vi "Compare Configs.vi"(10 "Old Config":path, 11 "New Config":path) -> (3 "Time":dbl)   [LabVIEW 2015]
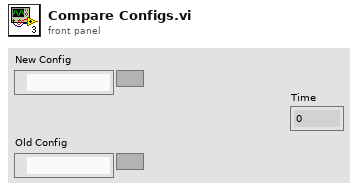
[diagram p1: front panel]
types:
  T1 = typedef "configuration.ctl" = cluster{"Primary Filter":string, "Secondary Filter":string, "Slit Mask":string, "Grating":string, "CS Target":dbl, "GS Target":dbl, "Coll Focus":i32, "Camera Focus":i32, "Name":string, "User":string, "Date":string, "Comment":string, "use Flexure Comp?":bool, "Select Mode:":u16}
  T2 = cluster{"Primary Filter":bool, "Secondary Filter":bool, "Slit Mask":bool, "Grating":bool, "CS Target":bool, "GS Target":bool, "Coll Focus":bool, "Camera Focus":bool, "Name":bool, "User":bool, "Date":bool, "Comment":bool, "use Flexure Comp?":bool, "Select Mode:":bool}
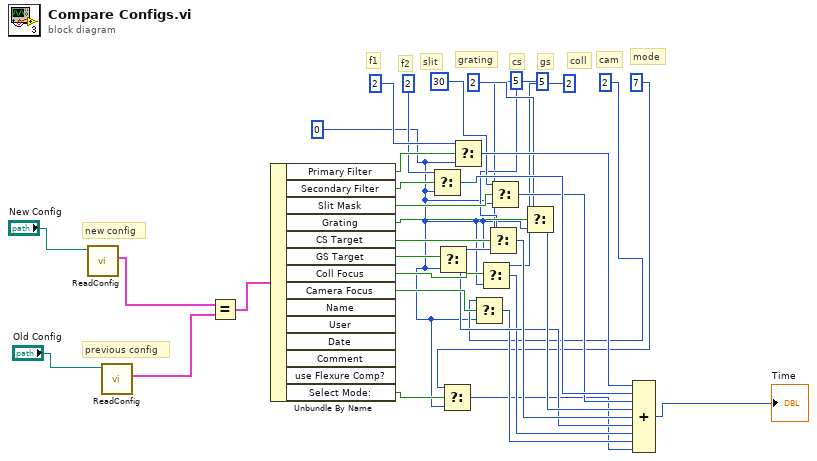
[diagram p0: block diagram]
diagram:
  w1 = 0
  # "mode"
  # "cam"
  # "coll"
  # "gs"
  # "cs"
  # "grating"
  # "slit"
  # "f2"
  # "f1"
  # "previous config"
  # "new config"
  n1 = call "ReadConfig.vi"("configuration file path"="New Config") -> ("Configuration"=w32:T1)  [unwired: 3 in, 3 out]
  n2 = call "ReadConfig.vi"("configuration file path"="Old Config") -> ("Configuration"=w31:T1)  [unwired: 3 in, 3 out]
  n3 = Equal?(x=w32, y=w31) -> (x = y?=w30:T2)
  n4 = Unbundle By Name(w30) -> ("Primary Filter"=w29:bool, "Secondary Filter"=w28:bool, "Slit Mask"=w27:bool, "Grating"=w26:bool, "CS Target"=w25:bool, "GS Target"=w24:bool, "Coll Focus"=w23:bool, "Camera Focus"=w22:bool, "Select Mode:"=w21:bool)  [unwired: 5 out]
  n5 = Select(t=2, s=w28, f=w1) -> (s? t:f=w18:i32)
  n6 = Select(t=5, s=w24, f=w1) -> (s? t:f=w14:i32)
  n7 = Select(t=7, s=w21, f=w1) -> (s? t:f=w11:i32)
  n8 = Select(t=2, s=w29, f=w1) -> (s? t:f=w19:i32)
  n9 = Select(t=2, s=w22, f=w1) -> (s? t:f=w12:i32)
  n10 = Select(t=2, s=w23, f=w1) -> (s? t:f=w13:i32)
  n11 = Select(t=5, s=w25, f=w1) -> (s? t:f=w15:i32)
  n12 = Select(t=30, s=w27, f=w1) -> (s? t:f=w17:i32)
  n13 = Select(t=2, s=w26, f=w1) -> (s? t:f=w16:i32)
  n14 = Compound Arithmetic op=ADD(w19, w18, w17, w16, w15, w14, w13, w12, w11) -> (→"Time":i32)
